vi "BRig_Host__Loop_Producer__tcp_System__Data_labelFiles_getExcelHandles.vi"() -> (0 "output_hExcel":bool, 1 "output_hExcel_Workbooks":refnum<k7>, 2 "output_hExcel_Application":refnum<k7>, 3 "output_excel_runningPreviously":bool, 6 "output_haveErrorMsg":string)   [LabVIEW 2014]
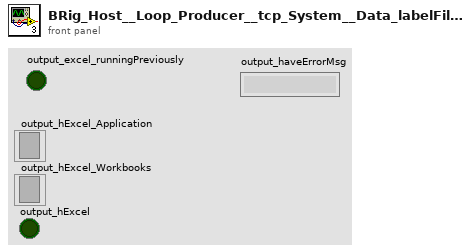
[diagram p1: front panel]
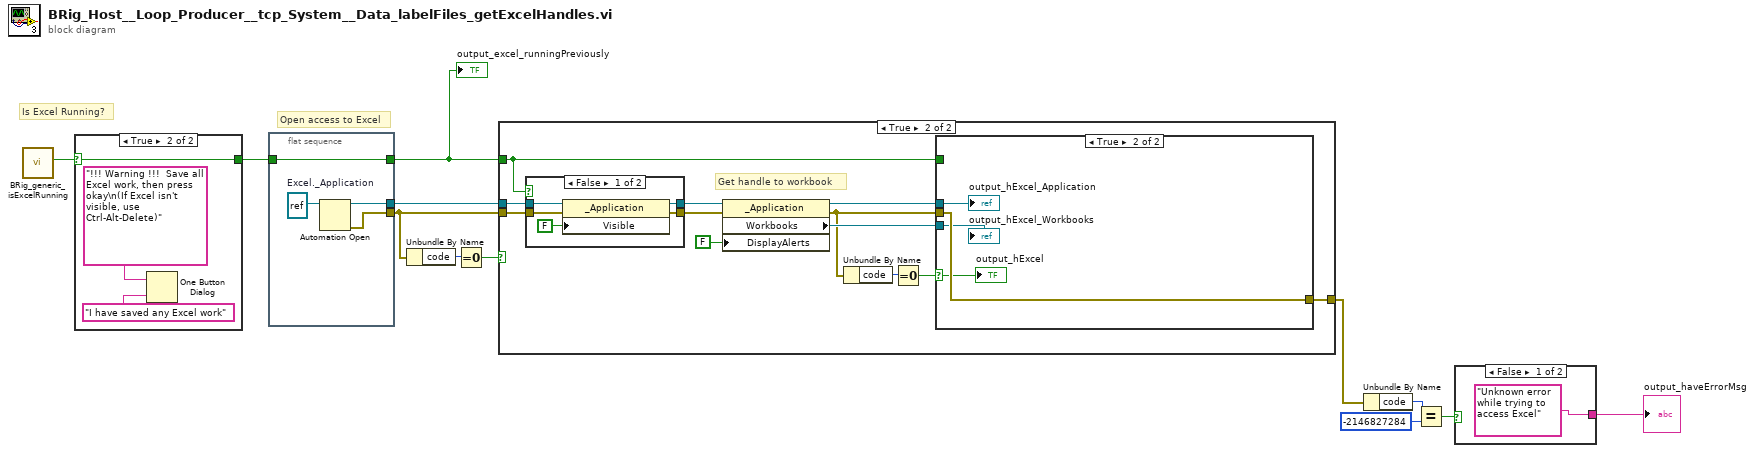
[diagram p0: block diagram]
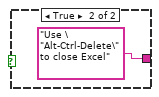
[diagram p2: hidden frame]
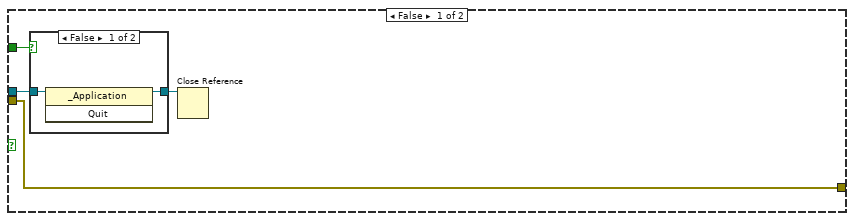
[diagram p3: hidden frame]
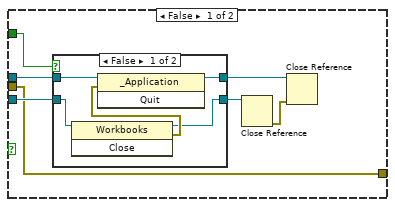
[diagram p5: hidden frame]
diagram:
  # "Open access to Excel"
  # "Is Excel Running?"
  n1 = call "BRig_generic_isExcelRunning.vi"() -> ("output_Iexcel"=w12:bool)  [unwired: 11 in]
  n2 = case shown="True" w12 {
    selector: w12 -> [w13 w14]
    tunnel: [w13 w14] -> w11
    frame False {
    }
    frame True {
      n3 = One Button Dialog(message="!!! Warning !!!  Save all Excel work, then press okay\n(If Excel isn't visible, use Ctrl-Alt-Delete)", button name ("OK")="I have saved any Excel work") -> ()  [unwired: 1 out]
    }
  }
  n4 = flat-sequence {
    tunnel: w11 -> [w19]
    tunnel: [w19] -> w8
    tunnel: [w18] -> w7
    tunnel: [w17] -> w6
    frame #0 {
      w20 = refnum<k7> refnum  # Excel._Application
      n5 = Automation Open(Automation Refnum=w20) -> (Automation Refnum=w18:refnum<k7>, error out=w17:errorcluster)  [unwired: 1 in, 2 out]
    }
  }
  n6 = Unbundle By Name(w6) -> ("code"=w10:i32)
  n7 = Equal To 0?(x=w10) -> (x = 0?=w9:bool)
  n8 = case shown="True" w9 {
    tunnel: w8 -> [w24 w31]
    tunnel: w7 -> [w23 w36]
    tunnel: w6 -> [w21 w35]
    tunnel: [w21 w28] -> w3
    frame False {
      n9 = case shown="False" w24 {
        tunnel: w23 -> [w26 w27]
        tunnel: [w25 w27] -> w22
        frame False {
          n10 = invoke class="_Application" method="Quit"(reference=w26) -> (reference out=w25:refnum<k7>)  [unwired: 2 in, 2 out]
        }
        frame True {
        }
      }
      n11 = Close Reference(reference=w22) -> ()  [unwired: 1 in, 1 out]
    }
    frame True {
      # "Get handle to workbook"
      n12 = case shown="False" w31 {
        tunnel: w36 -> [w61 w64]
        tunnel: w35 -> [w60 w63]
        tunnel: [w59 w63] -> w38
        tunnel: [w58 w64] -> w39
        frame False {
          n13 = property class="_Application"(reference=w61, error in=w60, "Visible"=FALSE) -> (reference out=w58:refnum<k7>, error out=w59:errorcluster)
        }
        frame True {
        }
      }
      n14 = property class="_Application"(reference=w39, error in=w38, "DisplayAlerts"=FALSE) -> (reference out=w33:refnum<k7>, error out=w29:errorcluster, "Workbooks"=w30:refnum<k7>)
      n15 = Unbundle By Name(w29) -> ("code"=w34:i32)
      n16 = Equal To 0?(x=w34) -> (x = 0?=w32:bool)
      n17 = case shown="True" w32 {
        selector: w32 -> [_ w54]
        tunnel: w33 -> [w45 w56]
        tunnel: w31 -> [w44 _]
        tunnel: w30 -> [w43 w55]
        tunnel: w29 -> [w40 w57]
        tunnel: [w40 w57] -> w28
        frame False {
          n18 = case shown="False" w44 {
            tunnel: w45 -> [w51 w53]
            tunnel: [w50 w53] -> w46
            tunnel: w43 -> [w49 w52]
            tunnel: [w47 w52] -> w42
            frame False {
              n19 = invoke class="Workbooks" method="Close"(reference=w49) -> (reference out=w47:refnum<k7>, error out=w48:errorcluster)  [unwired: 2 in, 1 out]
              n20 = invoke class="_Application" method="Quit"(reference=w51, error in=w48) -> (reference out=w50:refnum<k7>)  [unwired: 1 in, 2 out]
            }
            frame True {
            }
          }
          n21 = Close Reference(reference=w42) -> (error out=w41:errorcluster)  [unwired: 1 in]
          n22 = Close Reference(reference=w46, error in (no error)=w41) -> ()  [unwired: 1 out]
        }
        frame True {
          "output_hExcel_Application" <- w56
          "output_hExcel_Workbooks" <- w55
          "output_hExcel" <- w54
        }
      }
    }
  }
  n23 = Unbundle By Name(w3) -> ("code"=w4:i32)
  n24 = Equal?(x=w4, y=-2146827284) -> (x = y?=w1:bool)
  n25 = case shown="False" w1 {
    tunnel: ["Unknown error while trying to access Excel" ("message") "Use \"Alt-Ctrl-Delete\" to close Excel" ("message")] -> w2
    frame False {
    }
    frame True {
    }
  }
  "output_haveErrorMsg" <- w2
  "output_excel_runningPreviously" <- w8
